vi "Init Events.vi"(8 "error in (no error)":errorcluster, 11 "DiscoveryService in":refnum<class "NodeDiscovery.lvclass">) -> (0 "error out":errorcluster, 3 "DiscoveryService out":refnum<class "NodeDiscovery.lvclass">)   [LabVIEW 2020, in "Vecto.lvlib" / "NodeDiscovery.lvclass"]
uses:
  NodeDiscovery.lvclass
  NodeDiscovery.lvclass/NodeDiscovery.ctl
  Incoming Events.ctl
  proto/ServiceType/Enumeration.ctl
  proto/ServiceType/ServiceType.lvlib
  proto/Service/Data.ctl
  proto/Service/Service.lvlib
  Update Service Data.ctl
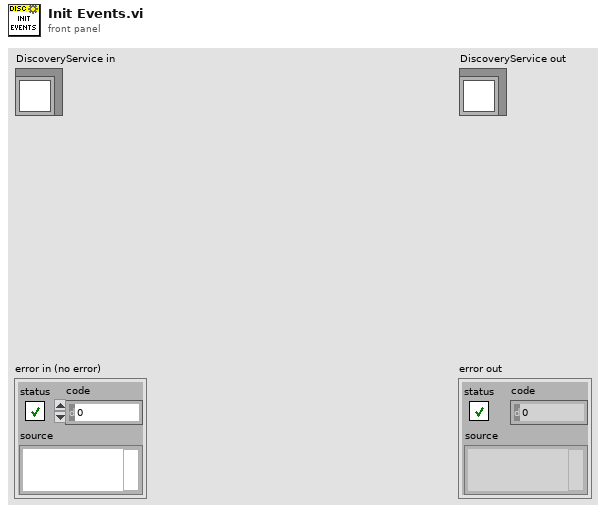
[diagram p1: front panel]
types:
  T1 = typedef "ServiceType.lvlib/Enumeration.ctl" = enum16{"SERVICETYPE_UNKNOWN", "SERVICETYPE_TCPSERVER", "SERVICETYPE_HTTPSERVER"}
  T2 = typedef "Vecto.lvlib/NodeDiscovery.lvclass/Update Service Data.ctl" = cluster{"Service":T3}
  T3 = typedef "Service.lvlib/Data.ctl" = cluster{"type":T1, "port":i32}
  T4 = typedef "Vecto.lvlib/NodeDiscovery.lvclass/Incoming Events.ctl" = cluster{"Close":refnum<user-event>, "Update Service":refnum<user-event>, "Update Status":refnum<user-event>, "Remove Service":refnum<user-event>, "Update Cfg Version":refnum<user-event>}
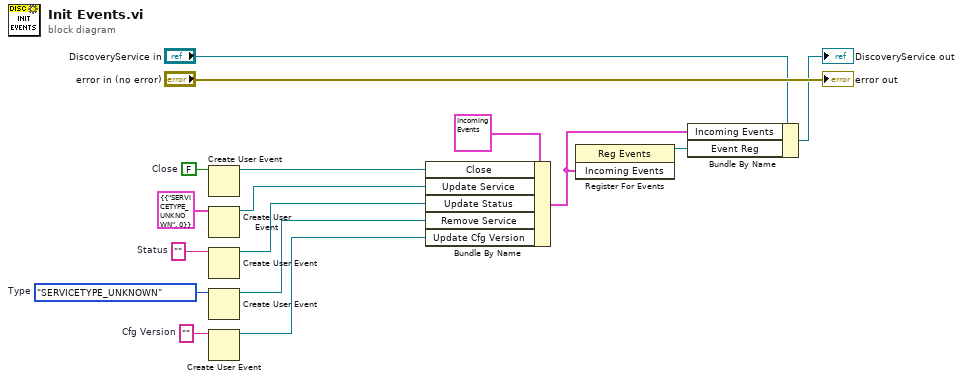
[diagram p0: block diagram]
diagram:
  w2 = ""  # Cfg Version
  w4 = Enumeration."SERVICETYPE_UNKNOWN"  # Type
  w6 = ""  # Status
  w15 = FALSE  # Close
  n1 = Create User Event(user event datatype=w15) -> (user event=w13:refnum<user-event>)  [unwired: 1 in, 1 out]
  n2 = Create User Event(user event datatype=T2 {"Service"={"type"=enum."SERVICETYPE_UNKNOWN", "port"=0}} ("Update Service Data")) -> (user event=w7:refnum<user-event>)  [unwired: 1 in, 1 out]
  n3 = Create User Event(user event datatype=w6) -> (user event=w5:refnum<user-event>)  [unwired: 1 in, 1 out]
  n4 = Create User Event(user event datatype=w4) -> (user event=w3:refnum<user-event>)  [unwired: 1 in, 1 out]
  n5 = Create User Event(user event datatype=w2) -> (user event=w1:refnum<user-event>)  [unwired: 1 in, 1 out]
  n6 = Bundle By Name(cluster=T4 {"Close"=refnum, "Update Service"=refnum, "Update Status"=refnum, "Remove Service"=refnum, "Update Cfg Version"=refnum} ("Incoming Events"), "Close"=w13, "Update Service"=w7, "Update Status"=w5, "Remove Service"=w3, "Update Cfg Version"=w1) -> (w11:T4)
  n7 = register-events(w11) -> (reference out=w10:refnum<event-registration>)  [unwired: 2 in, 1 out]
  n8 = Bundle By Name(cluster="DiscoveryService in", "Incoming Events"=w11, "Event Reg"=w10) -> (→"DiscoveryService out":refnum<class "NodeDiscovery.lvclass">)
  "error out" <- "error in (no error)"
